vi "Measure.vi"(8 "error in (no error)":errorcluster, 11 "Frequency Measurement in":refnum<class "Frequency Measurement.lvclass">) -> (0 "error out":errorcluster, 3 "Frequency Measurement out":refnum<class "Frequency Measurement.lvclass">)   [LabVIEW 2015, in "Frequency Measurement.lvlib" / "Frequency Measurement.lvclass"]
uses:
  Frequency Measurement.lvclass
  Results/Freq Result/Freq Sweep Result.lvclass
  <userlib>/Common Components/Measurement Actor/Measurement.lvclass/Measurement.ctl
  <userlib>/Common Components/Measurement Actor/Measurement.lvclass
  <userlib>/Common Components/Results/Results.lvclass
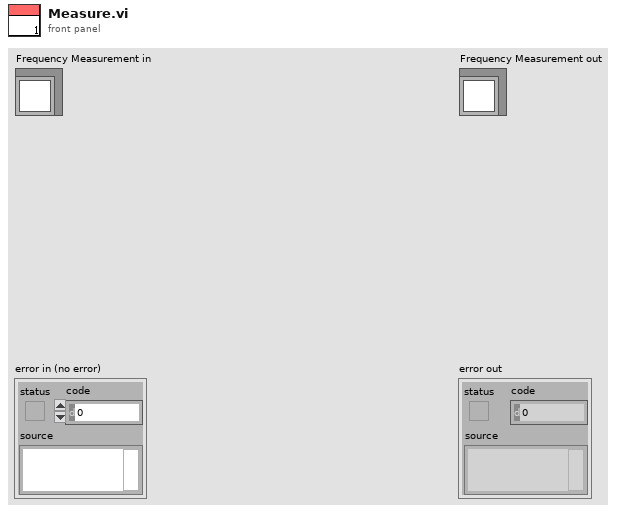
[diagram p1: front panel]
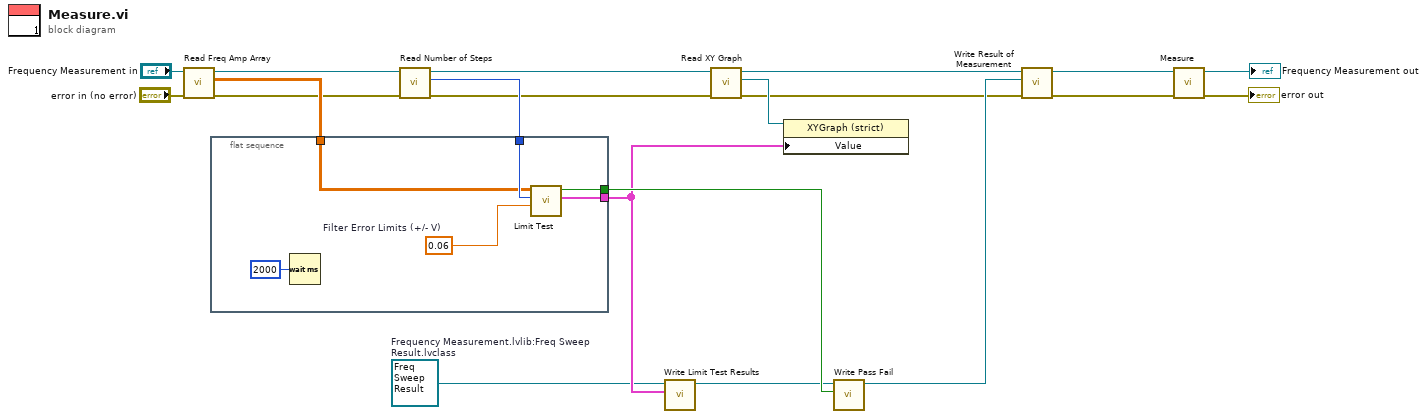
[diagram p0: block diagram]
diagram:
  w7 = refnum<class "Freq Sweep Result.lvclass"> refnum  # Frequency Measurement.lvlib:Freq Sweep Result.lvclass
  n1 = call "Read Freq Amp Array.vi"("error in (no error)"="error in (no error)", "Frequency Measurement in"="Frequency Measurement in") -> ("error out"=w15:errorcluster, "Freq Amp Array"=w19:dbl[][], "Frequency Measurement out"=w18:refnum<class "Frequency Measurement.lvclass">)  [unwired: 7 in]
  n2 = flat-sequence {
    tunnel: w20 -> [w25]
    tunnel: w19 -> [w24]
    tunnel: [w23] -> w11
    tunnel: [w22] -> w9
    frame #0 {
      w26 = 0.06  # Filter Error Limits (+/- V)
      n3 = Wait (ms)(milliseconds to wait=u32 2000) -> ()  [unwired: 1 out]
      n4 = call "Limit Test.vi"("Filter Error Limits"=w26, "Number of Steps"=w25, "Freq Amp Array"=w24) -> ("Limit Test Results"=w22:cluster{dbl[], dbl[]}[], "Test Passed?"=w23:bool)  [unwired: 2 in, 5 out]
    }
  }
  n5 = call "Read Number of Steps.vi"("error in (no error)"=w15, "Frequency Measurement in"=w18) -> ("error out"=w13:errorcluster, "Number of Steps"=w20:i32, "Frequency Measurement out"=w14:refnum<class "Frequency Measurement.lvclass">)  [unwired: 7 in]
  n6 = call "Write Limit Test Results.vi"("Limit Test Results"=w9, "Freq Sweet Result in"=w7) -> ("Freq Sweet Result out"=w10:refnum<class "Freq Sweep Result.lvclass">)  [unwired: 8 in, 1 out]
  n7 = call "Read XY Graph.vi"("error in (no error)"=w13, "Frequency Measurement in"=w14) -> ("error out"=w2:errorcluster, "XY Graph"=w12:refnum<vi>, "Frequency Measurement out"=w8:refnum<class "Frequency Measurement.lvclass">)  [unwired: 7 in]
  n8 = property class="XYGraph (strict)"(reference=w12, "Value"=w9) -> ()  [unwired: 1 in, 2 out]
  n9 = call <userlib>:"Write Pass Fail.vi"("Pass Fail"=w11, "Results in"=w10) -> ("Results out"=w3:refnum<class "Freq Sweep Result.lvclass">)  [unwired: 8 in, 1 out]
  n10 = call <userlib>:"Write Result of Measurement.vi"("error in (no error)"=w2, "Result Actor.lvlib:Results.lvclass"=w3, "Measurement in"=w8) -> ("error out"=w1:errorcluster, "Measurement out"=w4:refnum<class "Frequency Measurement.lvclass">)  [unwired: 7 in]
  n11 = call-parent "Measure.vi"("error in (no error)"=w1, "Measurement in"=w4) -> ("error out"=→"error out":errorcluster, "Measurement out"=→"Frequency Measurement out":refnum<class "Frequency Measurement.lvclass">)  [unwired: 8 in]
